vi "UsrProfiles-Window initialisation.vi"(9 "Access source":T1(ring), 11 "ctrl refs":T2) -> ()   [LabVIEW 2020]
uses:
  Typedefs/User login window refs.ctl
  Globals/gl_UsrProfiles globals.vi
  Global Variables/General Globals.vi
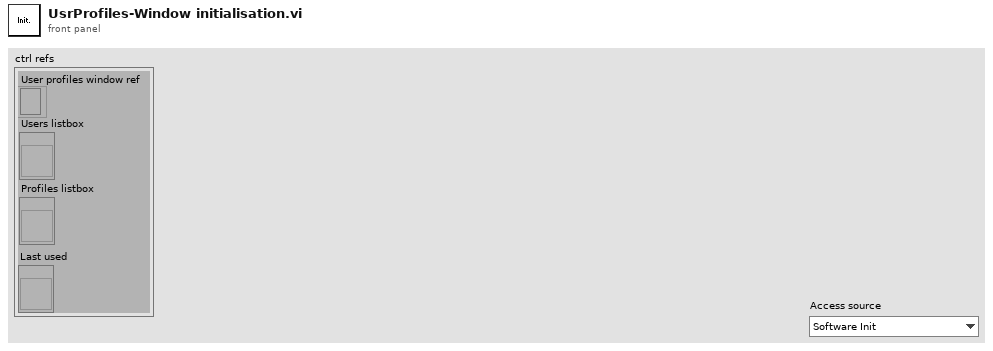
[diagram p1: front panel]
types:
  T1 = enum16{"Software Init", "User menu", "Switch User button"}
  T2 = typedef "User login window refs.ctl" = cluster{"User profiles window ref":refnum<k9>, "Users listbox":refnum<vi>, "Profiles listbox":refnum<vi>, "Last used":refnum<vi>}
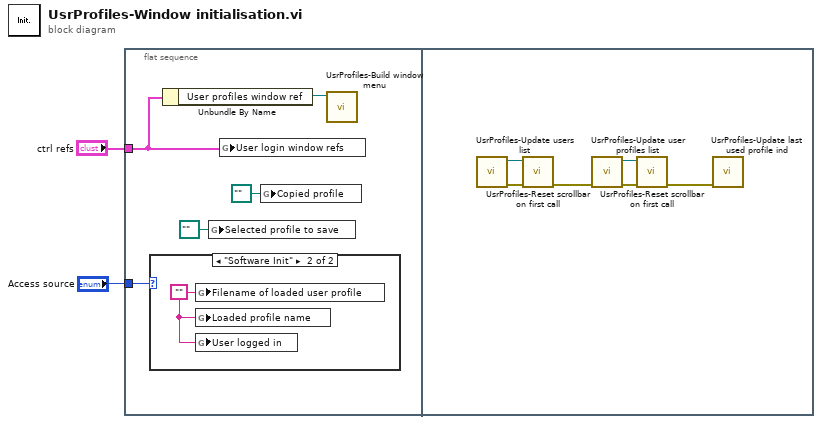
[diagram p0: block diagram]
diagram:
  n1 = flat-sequence {
    tunnel: "ctrl refs" -> [w4]
    tunnel: "Access source" -> [w5]
    frame #0 {
      n2 = case shown="\"Software Init\"" w5 {
        frame Default {
        }
        frame "Software Init" {
          w8 = "" ("Filename of loaded user profile")
          n3 = global write "General Globals.vi" "Filename of loaded user profile"(w8) -> ()
          n4 = global write "gl_UsrProfiles globals.vi" "Loaded profile name"(w8) -> ()
          n5 = global write "gl_UsrProfiles globals.vi" "User logged in"(w8) -> ()
        }
      }
      n6 = Unbundle By Name(w4) -> ("User profiles window ref"=w3:refnum<k9>)
      n7 = global write "gl_UsrProfiles globals.vi" "Selected profile to save"(path "" ("Copied profile")) -> ()
      n8 = global write "gl_UsrProfiles globals.vi" "User login window refs"(w4) -> ()
      n9 = global write "gl_UsrProfiles globals.vi" "Copied profile"(path "" ("Copied profile")) -> ()
      n10 = call "UsrProfiles-Build window menu.vi"("UsrProfiles-Window ref"=w3) -> ()  [unwired: 9 in, 2 out]
    }
    frame #1 {
      n11 = call "UsrProfiles-Update users list.vi"() -> ("error out"=w14:errorcluster, "Users listbox"=w12:refnum<vi>)  [unwired: 10 in]
      n12 = call "UsrProfiles-Reset scrollbar on first call.vi"("error in (no error)"=w14, "ListBox"=w12) -> ("error out"=w13:errorcluster)  [unwired: 9 in]
      n13 = call "UsrProfiles-Update user profiles list.vi"("error in"=w13) -> ("error out"=w10:errorcluster, "reference out"=w11:refnum<vi>)  [unwired: 9 in]
      n14 = call "UsrProfiles-Reset scrollbar on first call.vi"("error in (no error)"=w10, "ListBox"=w11) -> ("error out"=w9:errorcluster)  [unwired: 9 in]
      n15 = call "UsrProfiles-Update last used profile ind.vi"("error in"=w9) -> ()  [unwired: 10 in, 1 out]
    }
  }
